vi "SP_Correlation.vi"(9 "Tau Number":i64, 10 "New Count":dbl, 11 "initialize":bool) -> (1 "interation":i64, 3 "Cross Corr":dbl[](array[numeric]))   [LabVIEW 2022 SP3]
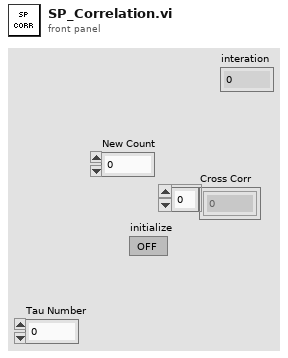
[diagram p1: front panel]
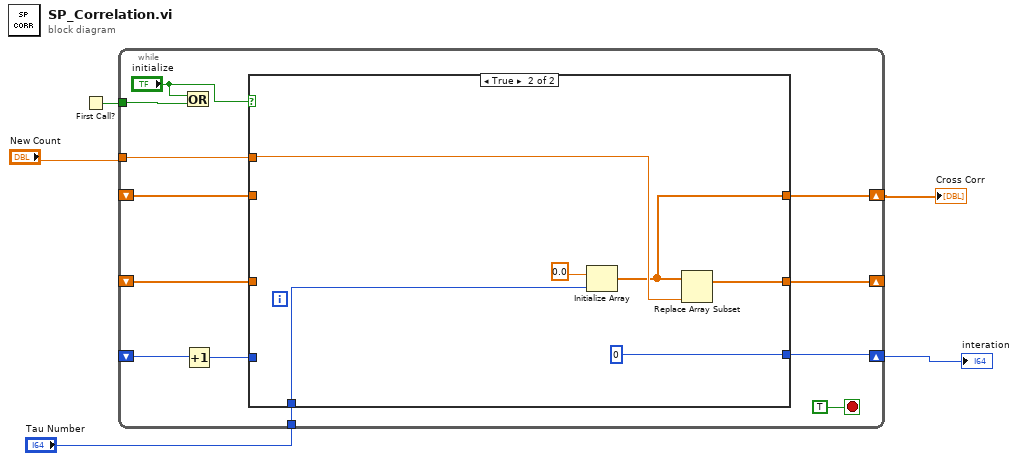
[diagram p0: block diagram]
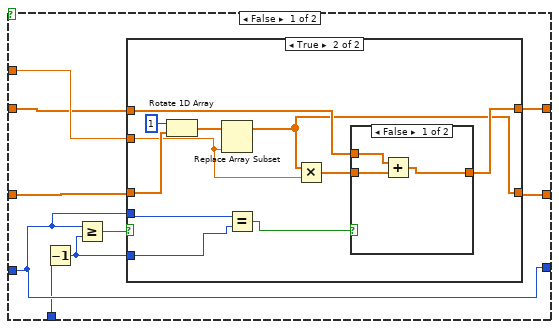
[diagram p2: hidden frame]
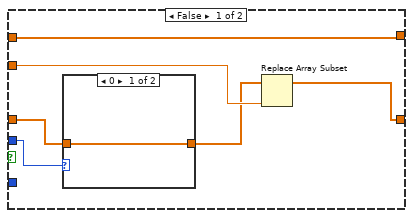
[diagram p3: hidden frame]
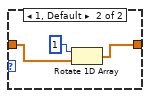
[diagram p4: hidden frame]
diagram:
  n1 = First Call?() -> (First Call?: T/F=w4:bool)
  n2 = while {
    tunnel: "New Count" -> [w15]
    shift-right: [w16] -> _
    shift-left: _ -> [w17]
    shift-right: [w14] -> w5
    shift-left: _ -> [w13]
    tunnel: w4 -> [w11]
    shift-right: [w10] -> w2
    shift-left: _ -> [w8]
    tunnel: "Tau Number" -> [w9]
    stop <- TRUE stop-if-true
    n3 = Or(x="initialize", y=w11) -> ()  [unwired: 1 out]
    n4 = Increment(x=w8) -> (x+1=w7:i32)
    n5 = case shown="True" "initialize" {
      tunnel: w17 -> [w26 _]
      tunnel: [w25 w54] -> w16
      tunnel: w15 -> [w24 w55]
      tunnel: [w22 w52] -> w14
      tunnel: w13 -> [w21 _]
      tunnel: [w20 0 ("Tau Number")] -> w10
      tunnel: w9 -> [w19 w53]
      tunnel: w7 -> [w20 _]
      frame False {
        n6 = Decrement(x=w19) -> (x-1=w18:i64)
        n7 = Greater Or Equal?(x=w20, y=w18) -> (x >= y?=w23:bool)
        n8 = case shown="True" w23 {
          tunnel: w24 -> [w32 w40]
          tunnel: w26 -> [w30 w47]
          tunnel: [w28 w41] -> w25
          tunnel: [w27 w44] -> w22
          tunnel: w21 -> [w27 w43]
          tunnel: w20 -> [w31 w39]
          tunnel: w18 -> [_ w37]
          frame False {
            n9 = case shown="0" w31 {
              tunnel: w30 -> [w33 w35]
              tunnel: [w33 w34] -> w29
              frame 0 {
              }
              frame 1, Default {
                n10 = Rotate 1D Array(1:w35, 2:1 ("n")) -> (0:w34:dbl[])
              }
            }
            n11 = Replace Array Subset(array=w29, new element=w32) -> (w28:dbl[])  [unwired: 1 in]
          }
          frame True {
            n12 = Rotate 1D Array(1:w47, 2:1 ("n")) -> (0:w45:dbl[])
            n13 = Replace Array Subset(array=w45, new element=w40) -> (w41:dbl[])  [unwired: 1 in]
            n14 = Equal?(x=w39, y=w37) -> (x = y?=w38:bool)
            n15 = Multiply(x=w41, y=w40) -> (x*y=w46:dbl[])
            n16 = case shown="False" w38 {
              tunnel: w46 -> [w50 w51]
              tunnel: [w48 w51] -> w44
              tunnel: w43 -> [w49 _]
              frame False {
                n17 = Add(x=w49, y=w50) -> (x+y=w48:dbl[])
              }
              frame True {
              }
            }
          }
        }
      }
      frame True {
        n18 = Initialize Array(0.0 ("dimension size"), w53) -> (w52:dbl[])
        n19 = Replace Array Subset(array=w52, new element=w55) -> (w54:dbl[])  [unwired: 1 in]
      }
    }
  }
  "Cross Corr" <- w5
  "interation" <- w2
